vi "getConfig.vi"(8 "error in (no error)":errorcluster) -> (0 "error out":errorcluster, 3 "Config":T1)   [LabVIEW 2010, in "TPVG_DLL.lvlib"]
doc: "------------------------------------------\nAuthor: Dang Lam\nEmail: danglamtd@gmail.com"
uses:
  TPVG_DLL.lvlib
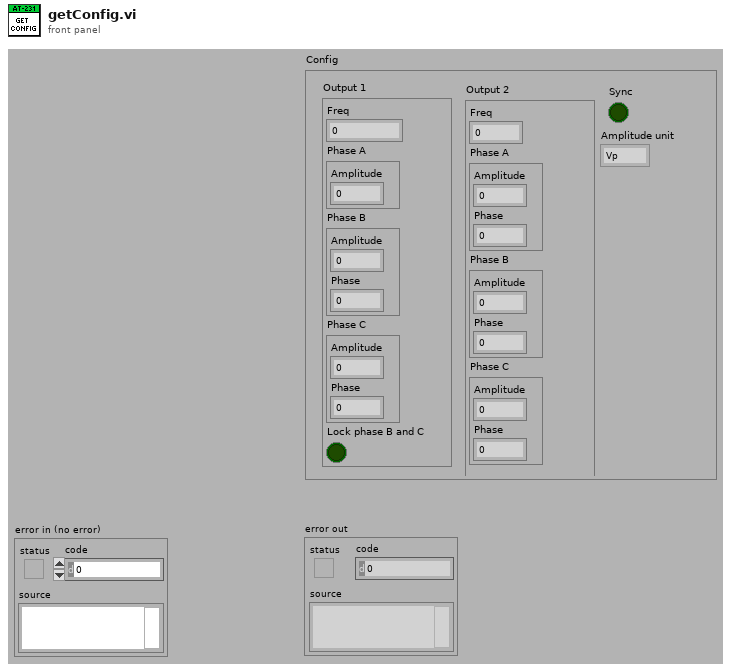
[diagram p1: front panel]
types:
  T1 = cluster{"Output 1":cluster{"Freq":sgl, "Phase A":cluster{"Amplitude":sgl}, "Phase B":cluster{"Amplitude":sgl, "Phase":sgl}, "Phase C":cluster{"Amplitude":sgl, "Phase":sgl}, "Lock":bool}, "Output 2":cluster{"Freq":sgl, "Phase A":cluster{"Amplitude":sgl, "Phase":sgl}, "Phase B":cluster{"Amplitude":sgl, "Phase":sgl}, "Phase C":cluster{"Amplitude":sgl, "Phase":sgl}, "Lock":bool}, "Sync":bool, "Amplitude unit":enum16{"Vp", "Vp-p", "Vrms"}}
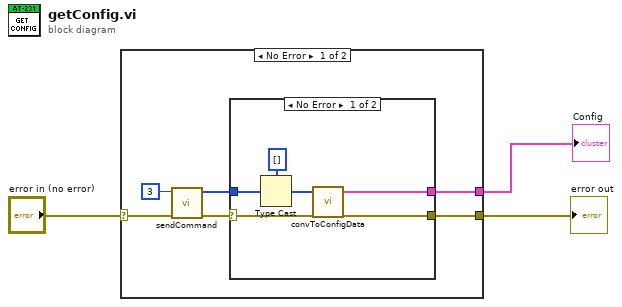
[diagram p0: block diagram]
diagram:
  n1 = case shown="No Error" "error in (no error)" {
    selector: "error in (no error)" -> [w9 w16]
    tunnel: [w6 w16] -> w2
    tunnel: [w4 _] -> w1
    frame No Error {
      n2 = call "sendCommand.vi"("error in (no error)"=w9, "Command ID"=u16 3) -> ("error out"=w7:errorcluster, "Data out"=w5:u8[])  [unwired: 8 in]
      n3 = case shown="No Error" w7 {
        selector: w7 -> [w14 w15]
        tunnel: [w14 w15] -> w6
        tunnel: w5 -> [w13 _]
        tunnel: [w10 _] -> w4
        frame No Error {
          n4 = Type Cast(type=u16[] [], x=w13) -> (*(type *) &x=w11:u16[])
          n5 = call "convToConfigData.vi"("Raw Config in"=w11) -> ("Config out"=w10:T1)  [unwired: 4 in]
        }
        frame Error {
        }
      }
    }
    frame Error {
    }
  }
  "error out" <- w2
  "Config" <- w1
